vi "Test Optimized Flatten Unflatten.vi"() -> ()   [LabVIEW 2021]
uses:
  Endian.ctl
  DataTypes_CIF_U.lvlib
panel:
  out "Pass":bool
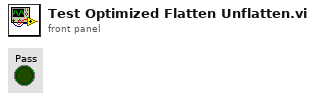
[diagram p1: front panel]
types:
  T1 = enum16{"big-endian, network order", "native, host order", "little-endian"}
  T2 = typedef "DataTypes_CIF_U.lvlib/Endian.ctl" = enum16{"Little Endian", "Big Endian"}
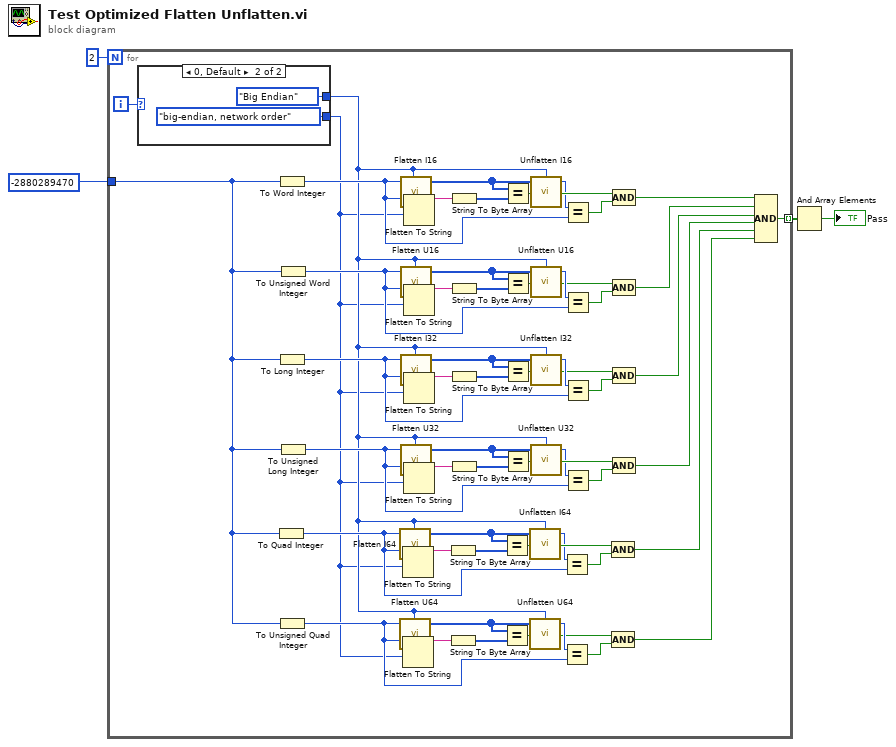
[diagram p0: block diagram]
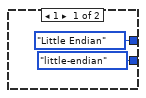
[diagram p2: hidden frame]
diagram:
  n1 = for {
    N: 2 -> [_]
    tunnel: [w57] -> w4 mode=indexing
    tunnel: i64 -2880289470 ("i16") -> [w10]
    i -> [w54]
    n2 = case shown="0, Default" w54 {
      tunnel: [T1."little-endian" ("byte order (0:big-endian, network order)") T1."big-endian, network order" ("byte order (0:big-endian, network order)")] -> w11
      tunnel: [Endian."Little Endian" ("Endian") Endian."Big Endian" ("Endian")] -> w12
      frame 1 {
      }
      frame 0, Default {
      }
    }
    n3 = To Quad Integer(1:w10) -> (0:w41:i64)
    n4 = To Word Integer(number=w10) -> (16bit integer=w13:i16)
    n5 = To Long Integer(number=w10) -> (32bit integer=w40:i32)
    n6 = To Unsigned Quad Integer(1:w10) -> (0:w51:u64)
    n7 = To Unsigned Word Integer(number=w10) -> (unsigned 16bit integer=w22:u16)
    n8 = To Unsigned Long Integer(number=w10) -> (unsigned 32bit integer=w31:u32)
    n9 = call "Flatten I64.vi"("I64"=w41, "Endian"=w12) -> ("Flat Data"=w44:u8[])  [unwired: 3 in]
    n10 = call "Flatten U64.vi"("U64"=w51, "Endian"=w12) -> ("Flat Data"=w53:u8[])  [unwired: 3 in]
    n11 = call "Flatten I16.vi"("I16"=w13, "Endian"=w12) -> ("Flat Data"=w16:u8[])  [unwired: 3 in]
    n12 = call "Flatten U16.vi"("U16"=w22, "Endian"=w12) -> ("Flat Data"=w24:u8[])  [unwired: 3 in]
    n13 = call "Flatten I32.vi"("I32"=w40, "Endian"=w12) -> ("Flat Data"=w37:u8[])  [unwired: 3 in]
    n14 = call "Flatten U32.vi"("U32"=w31, "Endian"=w12) -> ("Flat Data"=w29:u8[])  [unwired: 3 in]
    n15 = Flatten To String(anything=w41, byte order (0:big-endian, network order)=w11) -> (data string=w42:string)  [unwired: 2 in, 2 out]
    n16 = Flatten To String(anything=w51, byte order (0:big-endian, network order)=w11) -> (data string=w56:string)  [unwired: 2 in, 2 out]
    n17 = Flatten To String(anything=w13, byte order (0:big-endian, network order)=w11) -> (data string=w14:string)  [unwired: 2 in, 2 out]
    n18 = Flatten To String(anything=w22, byte order (0:big-endian, network order)=w11) -> (data string=w26:string)  [unwired: 2 in, 2 out]
    n19 = Flatten To String(anything=w40, byte order (0:big-endian, network order)=w11) -> (data string=w39:string)  [unwired: 2 in, 2 out]
    n20 = Flatten To String(anything=w31, byte order (0:big-endian, network order)=w11) -> (data string=w27:string)  [unwired: 2 in, 2 out]
    n21 = String To Byte Array(string=w42) -> (unsigned byte array=w43:u8[])
    n22 = String To Byte Array(string=w56) -> (unsigned byte array=w55:u8[])
    n23 = String To Byte Array(string=w14) -> (unsigned byte array=w15:u8[])
    n24 = String To Byte Array(string=w26) -> (unsigned byte array=w25:u8[])
    n25 = String To Byte Array(string=w39) -> (unsigned byte array=w38:u8[])
    n26 = String To Byte Array(string=w27) -> (unsigned byte array=w28:u8[])
    n27 = Equal?(x=w44, y=w43) -> (x = y?=w47:bool)
    n28 = Equal?(x=w53, y=w55) -> (x = y?=w49:bool)
    n29 = Equal?(x=w16, y=w15) -> (x = y?=w19:bool)
    n30 = Equal?(x=w24, y=w25) -> (x = y?=w20:bool)
    n31 = Equal?(x=w37, y=w38) -> (x = y?=w34:bool)
    n32 = Equal?(x=w29, y=w28) -> (x = y?=w33:bool)
    n33 = call "Unflatten I64.vi"("Flat Data"=w44, "Endian"=w12) -> ("I64"=w45:i64)  [unwired: 3 in]
    n34 = call "Unflatten U64.vi"("Flat Data"=w53, "Endian"=w12) -> ("U64"=w52:u64)  [unwired: 3 in]
    n35 = call "Unflatten I16.vi"("Flat Data"=w16, "Endian"=w12) -> ("I16"=w17:i16)  [unwired: 3 in]
    n36 = call "Unflatten U16.vi"("Flat Data"=w24, "Endian"=w12) -> ("U16"=w23:u16)  [unwired: 3 in]
    n37 = call "Unflatten I32.vi"("Flat Data"=w37, "Endian"=w12) -> ("I32"=w36:i32)  [unwired: 3 in]
    n38 = call "Unflatten U32.vi"("Flat Data"=w29, "Endian"=w12) -> ("U32"=w30:u32)  [unwired: 3 in]
    n39 = Equal?(x=w45, y=w41) -> (x = y?=w46:bool)
    n40 = Equal?(x=w52, y=w51) -> (x = y?=w50:bool)
    n41 = Equal?(x=w17, y=w13) -> (x = y?=w18:bool)
    n42 = Equal?(x=w23, y=w22) -> (x = y?=w21:bool)
    n43 = Equal?(x=w36, y=w40) -> (x = y?=w35:bool)
    n44 = Equal?(x=w30, y=w31) -> (x = y?=w32:bool)
    n45 = Compound Arithmetic op=AND(w47, w46) -> (w9:bool)
    n46 = Compound Arithmetic op=AND(w49, w50) -> (w48:bool)
    n47 = Compound Arithmetic op=AND(w19, w18) -> (w5:bool)
    n48 = Compound Arithmetic op=AND(w20, w21) -> (w6:bool)
    n49 = Compound Arithmetic op=AND(w34, w35) -> (w7:bool)
    n50 = Compound Arithmetic op=AND(w33, w32) -> (w8:bool)
    n51 = Compound Arithmetic op=AND(w5, w6, w7, w8, w9, w48) -> (w57:bool)
  }
  n52 = And Array Elements(Boolean array=w4) -> (logical AND=→"Pass":bool)
